vi "Find index of value in an array closest to target value.vi"(9 "start searching index":i32, 10 "Target value":dbl=4.2, 11 "Array":dbl[](array[numeric])=[1.0, 1.5, 2.0, 33.0, 4.0, 4.1, 4.3, 4.7, 7.0]) -> (2 "Closest value":dbl=4.3, 3 "Index of closest value":i32=6)   [LabVIEW 2016]
panel:
  out "Smallest difference (abs value)":dbl=0.09999999999999964
  # "This is where you start searching for the value closest to the target."
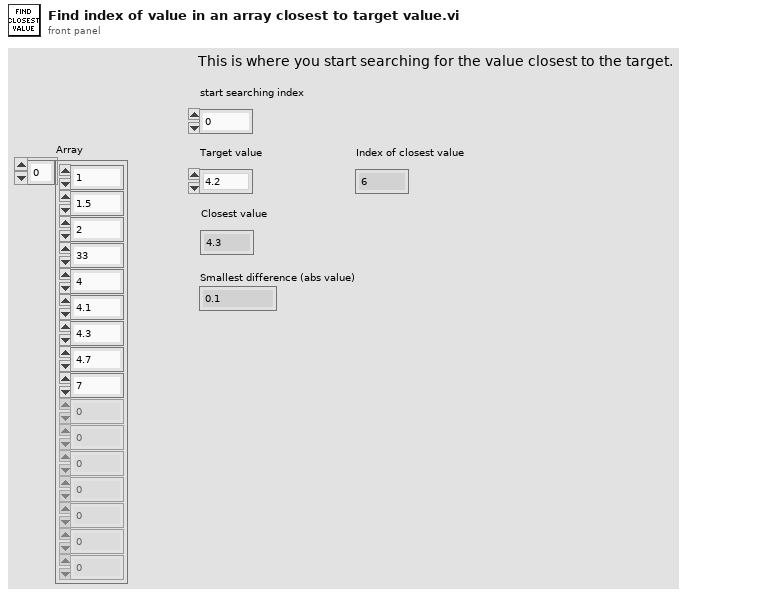
[diagram p1: front panel]
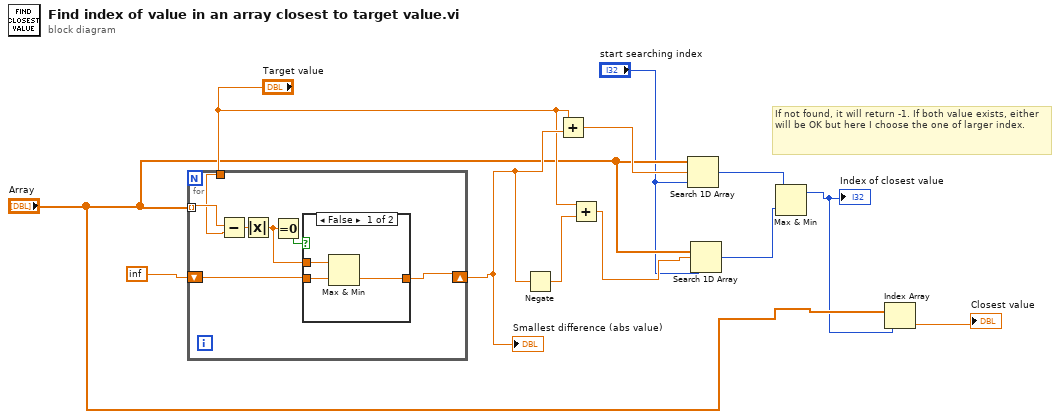
[diagram p0: block diagram]
diagram:
  # "If not found, it will return -1. If both value exists, either will be OK but here I choose the one of larger index."
  n1 = for {
    tunnel: "Array" -> [w15] mode=indexing
    shift-right: [w14] -> w9
    shift-left: inf -> [w19]
    tunnel: "Target value" -> [w13]
    n2 = Subtract(x=w15, y=w13) -> (x-y=w18:dbl)
    n3 = Absolute Value(x=w18) -> (abs(x)=w16:dbl)
    n4 = Equal To 0?(x=w16) -> (x = 0?=w17:bool)
    n5 = case shown="False" w17 {
      tunnel: w19 -> [w22 _]
      tunnel: [w21 w23] -> w14
      tunnel: w16 -> [w20 w23]
      frame False {
        n6 = Max & Min(x=w20, y=w22) -> (min(x,y)=w21:dbl)  [unwired: 1 out]
      }
      frame True {
      }
    }
  }
  "Smallest difference (abs value)" <- w9
  n7 = Negate(x=w9) -> (-x=w6:dbl)
  n8 = Add(x="Target value", y=w9) -> (x+y=w8:dbl)
  n9 = Add(x="Target value", y=w6) -> (x+y=w5:dbl)
  n10 = Search 1D Array(1D array="Array", element=w8, start index (0)="start searching index") -> (index of element=w11:i32)
  n11 = Search 1D Array(1D array="Array", element=w5, start index (0)="start searching index") -> (index of element=w10:i32)
  n12 = Max & Min(x=w11, y=w10) -> (max(x,y)=w3:i32)  [unwired: 1 out]
  "Index of closest value" <- w3
  n13 = Index Array(array="Array", index=w3) -> (element=→"Closest value":dbl)
